vi "AutoAlign_P541_V2.vi"() -> ()   [LabVIEW 2014]
uses:
  Controls/StageStates.ctl
  Controls/GraphNotifier2D.ctl
panel:
  out "Current Step":i32
  in  "Done":bool
  in  "Repeat":bool
  in  "Start":bool
  out "Cursor Position":dbl=40.46
  in  "InitialStep":dbl=-0.5
  in  "StepSize":dbl=0.03
  in  "Number Of Steps":i32=45
  out "Intensity Graph":sgl[][](graph)=[[1726.0, 1806.0, 1623.0, 1740.0, 1902.0, 2025.0, 2061.0, 2397.0, 1982.0, 2142.0, 1921.0, 1825.0, 1807.0, 1676.0, 1719.0], [1834.0, 1961.0, 1598.0, 2017.0, 2102.0, 2328.0, 2583.0, 2454.0, 2515.0, 2699.0, 2220.0, 2038.0, 1897.0, 1896.0, 1808.0], [1796.0, 1929.0, 2014.0, 2227.0, 2672.0, 3226.0, 3334.0, 3386.0, 3268.0, 2996.0, 2332.0, 2163.0, 1901.0, 1735.0, 1698.0], [1808.0, 2338.0, 2431.0, 2752.0, 3453.0, 4017.0, 4563.0, 4369.0, 4047.0, 3273.0, 2724.0, 2242.0, 2046.0, 1830.0, 1856.0], [1912.0, 2124.0, 3081.0, 2979.0, 5386.0, 11058.0, 13706.0, 11119.0, 6549.0, 3853.0, 2769.0, 2421.0, 1921.0, 1945.0, 1667.0], [1802.0, 2329.0, 2974.0, 5101.0, 13243.0, 29557.0, 37323.0, 29866.0, 11701.0, 4217.0, 2995.0, 2488.0, 2124.0, 2138.0, 1748.0], [1855.0, 2667.0, 2858.0, 6518.0, 22689.0, 47134.0, 57757.0, 40932.0, 16892.0, 4794.0, 2975.0, 2648.0, 2316.0, 1940.0, 2196.0], [1840.0, 2513.0, 2969.0, 6113.0, 20925.0, 44575.0, 52306.0, 35893.0, 13438.0, 3959.0, 2980.0, 2333.0, 2128.0, 1717.0, 1820.0], [1975.0, 2578.0, 2513.0, 4337.0, 10762.0, 22714.0, 27719.0, 17796.0, 6495.0, 3198.0, 2732.0, 2148.0, 1973.0, 1982.0, 1689.0], [1678.0, 2147.0, 2574.0, 2995.0, 4337.0, 7306.0, 8045.0, 5820.0, 3423.0, 2628.0, 2656.0, 2059.0, 2116.0, 1972.0, 1626.0], [1892.0, 2079.0, 2546.0, 2756.0, 2841.0, 3166.0, 3141.0, 2947.0, 2684.0, 2415.0, 1923.0, 1806.0, 2081.0, 1695.0, 1756.0], [1617.0, 1885.0, 1958.0, 2510.0, 2675.0, 2479.0, 2435.0, 2624.0, 2645.0, 2107.0, 1819.0, 2019.0, 1839.0, 1623.0, 1670.0], [1609.0, 1896.0, 1887.0, 1962.0, 2214.0, 2352.0, 2290.0, 2047.0, 1815.0, 2022.0, 1883.0, 1801.0, 1521.0, 1615.0, 1723.0], [1697.0, 1808.0, 1977.0, 1969.0, 2042.0, 1988.0, 2305.0, 2063.0, 1959.0, 1814.0, 1844.0, 1590.0, 1578.0, 1755.0, 1573.0], [1645.0, 1684.0, 1821.0, 1765.0, 1973.0, 1906.0, 2005.0, 1822.0, 1736.0, 1850.0, 1649.0, 1802.0, 1476.0, 1658.0, 1637.0]]
  in  "Quit":bool
  out "Sample":cluster{dbl[], dbl[]}[](graph)
  in  "Accumulations":i32=10
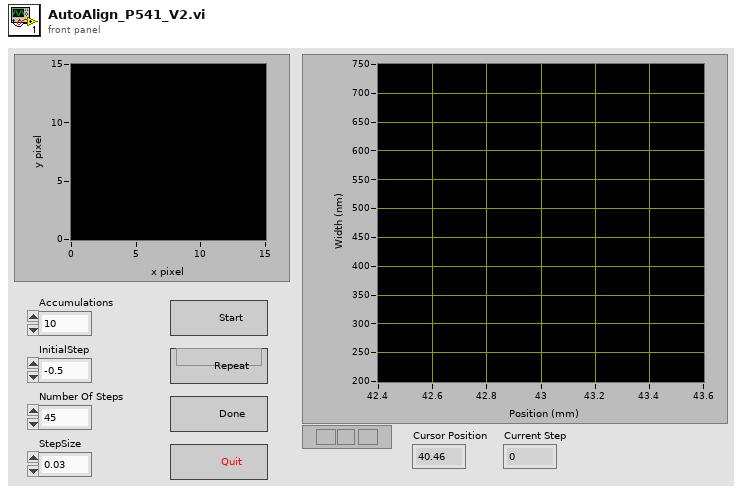
[diagram p1: front panel]
types:
  T1 = typedef "GraphNotifier2D.ctl" = cluster{"Xpos":i32, "Ypos":i32, "subarray":sgl[][], "Intensity":sgl}
  T2 = typedef "LabVIEW Interface for Arduino.lvlib/Arduino Resource.ctl" = cluster{"VISA resource":refnum<visa-resource-name>, "Board Type":T3, "Connection Type":enum8{"USB / Serial"}, "Bytes Per Packet (15)":u8}
  T3 = typedef "LabVIEW Interface for Arduino.lvlib/Board Type.ctl" = enum16{"Uno", "Dimuelanove w/Atmega 328", "Mega 2560"}
  T4 = typedef "StageStates.ctl" = enum16{"POSITION", "MVR", "MOVE", "HALT", "ONTARGET", "ERROR", "EXIT", "HOME", "ZEROPOS", "NANOPOS", "QUIT", "ANALOG"}
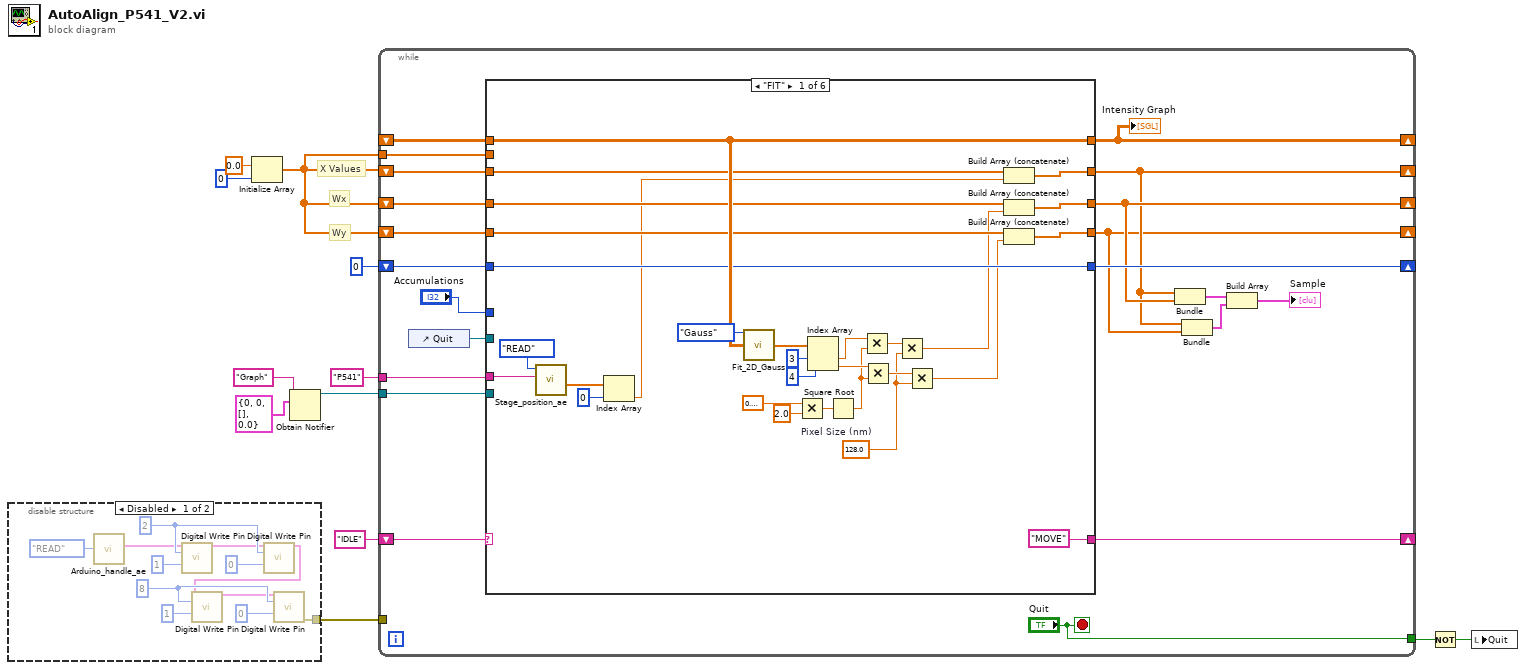
[diagram p0: block diagram]
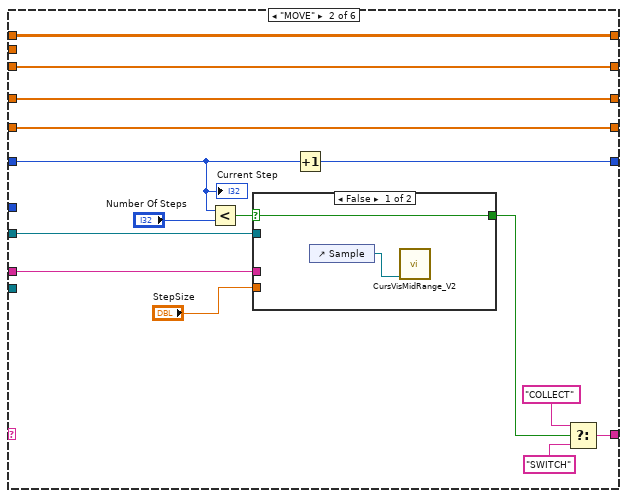
[diagram p3: hidden frame]
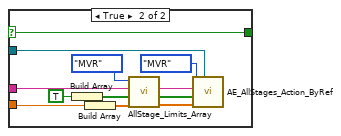
[diagram p4: hidden frame]
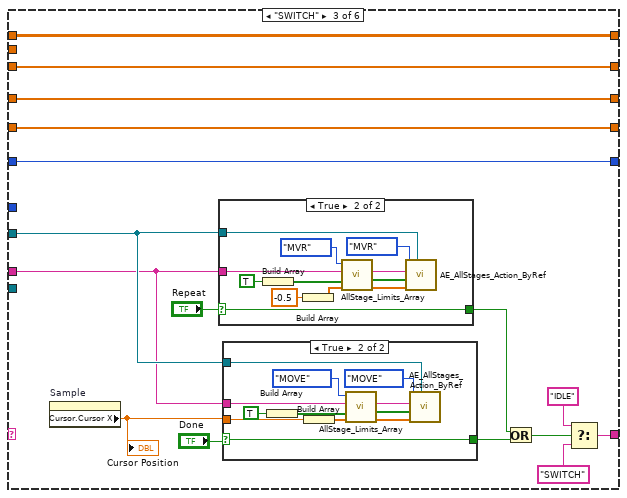
[diagram p5: hidden frame]
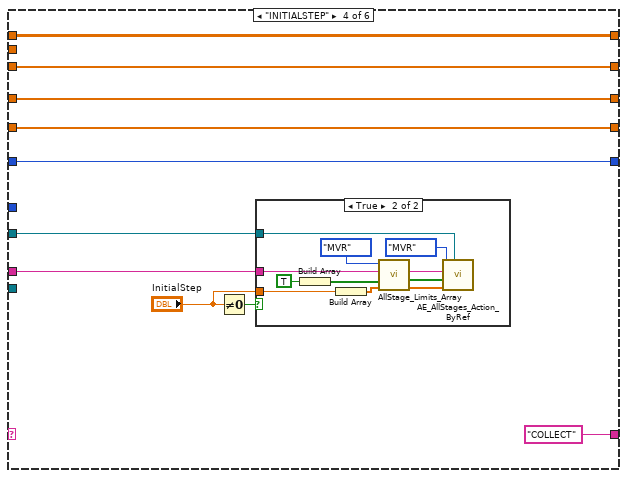
[diagram p8: hidden frame]
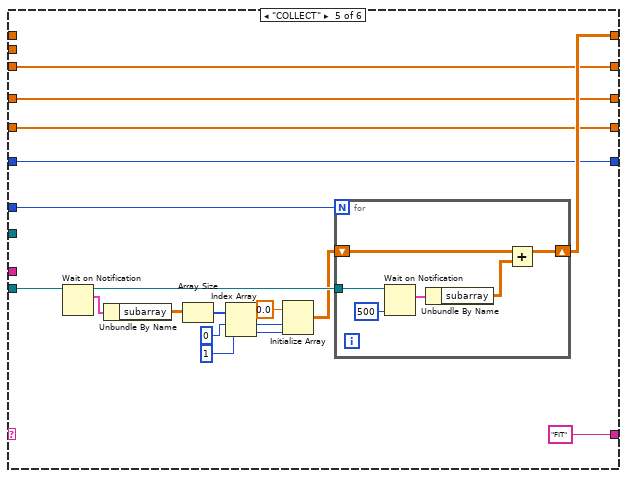
[diagram p10: hidden frame]
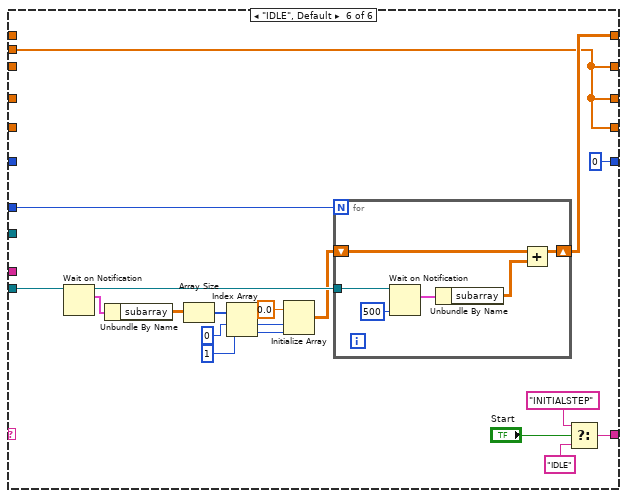
[diagram p11: hidden frame]
diagram:
  # "Wy"
  # "Wx"
  # "X Values"
  n1 = disable-structure shown="Disabled" {
    disable-tunnel: [w13 _] -> w9
    frame Disabled {
      w24 = u8 8 ("Digital I/O Pin (0)")
      w19 = u8 2 ("Digital I/O Pin (0)")
      n2 = call "Arduino_handle_ae.vi"("Enum"=enum16{"WRITE", "READ"}."READ") -> ("Arduino Resource Out"=w18:T2)  [unwired: 10 in]
      n3 = call <vilib>:"Digital Write Pin.vi"("Arduino Resource"=w18, "Digital I/O Pin (0)"=w19, "Value (0)"=u8 1) -> ("Arduino Resource"=w14:T2)  [unwired: 11 in, 1 out]
      n4 = call <vilib>:"Digital Write Pin.vi"("Arduino Resource"=w14, "Digital I/O Pin (0)"=w19, "Value (0)"=u8 0) -> ("Arduino Resource"=w23:T2)  [unwired: 11 in, 1 out]
      n5 = call <vilib>:"Digital Write Pin.vi"("Arduino Resource"=w23, "Digital I/O Pin (0)"=w24, "Value (0)"=u8 1) -> ("Arduino Resource"=w22:T2)  [unwired: 11 in, 1 out]
      n6 = call <vilib>:"Digital Write Pin.vi"("Arduino Resource"=w22, "Digital I/O Pin (0)"=w24, "Value (0)"=u8 0) -> ("error out"=w13:errorcluster)  [unwired: 11 in, 1 out]
    }
    frame Enabled {
    }
  }
  n7 = Initialize Array(0.0 ("element"), 0 ("dimension size")) -> (w1:dbl[])
  n8 = Obtain Notifier(name (unnamed)="Graph", notification data type=T1 {"Xpos"=0, "Ypos"=0, "subarray"=[], "Intensity"=0.0}) -> (notifier out=w6:refnum<notifier>)  [unwired: 2 in, 2 out]
  n9 = while {
    shift-right: [w44] -> _
    shift-left: _ -> [w45]
    shift-right: [w29] -> _
    shift-left: w1 -> [w35]
    shift-right: [w43] -> _
    shift-left: "IDLE" -> [w39]
    shift-right: [w41] -> _
    shift-left: 0 ("NumberOfSteps 2") -> [w42]
    tunnel: w6 -> [w38]
    tunnel: "P541" ("StageID") -> [w36]
    tunnel: w9 -> [_]
    tunnel: ["Quit"] -> w5
    shift-right: [w30] -> _
    shift-left: w1 -> [w33]
    shift-right: [w28] -> _
    shift-left: w1 -> [w32]
    tunnel: w1 -> [w31]
    stop <- "Quit" stop-if-true
    n10 = control-ref of="Quit"() -> (w40:refnum<vi>)
    n11 = case shown="\"FIT\"" w39 {
      tunnel: [w73 w89 w118 w155 w184 w209] -> w44
      tunnel: w45 -> [w73 w89 w118 w155 _ _]
      tunnel: w35 -> [w54 w77 w106 w148 w169 _]
      tunnel: w36 -> [w70 w80 w115 w151 _ _]
      tunnel: ["MOVE" w86 w112 "COLLECT" "FIT" w207] -> w43
      tunnel: w42 -> [w71 w84 w119 w154 w183 _]
      tunnel: [w71 w85 w119 w154 w183 0 ("NumberOfSteps 2")] -> w41
      tunnel: w40 -> [_ w82 w117 w153 _ _]
      tunnel: w38 -> [_ _ _ _ w172 w201]
      tunnel: "Accumulations" -> [_ _ _ _ w181 w204]
      tunnel: w33 -> [w52 w76 w105 w147 w168 _]
      tunnel: w32 -> [w53 w75 w104 w146 w167 _]
      tunnel: [w51 w77 w106 w148 w169 w191] -> w29
      tunnel: [w50 w76 w105 w147 w168 w191] -> w30
      tunnel: [w49 w75 w104 w146 w167 w191] -> w28
      tunnel: w31 -> [_ _ _ _ _ w191]
      frame "FIT" {
        w55 = 128.0  # Pixel Size (nm)
        n12 = call "Stage_position_ae.vi"("StageID"=w70, "Enum"=enum16{"WRITE", "READ"}."READ") -> ("Position Out"=w63:dbl[])  [unwired: 8 in, 1 out]
        n13 = Index Array(array=w63, index=0) -> (element=w48:dbl)
        n14 = call "Fit_2D_Gauss.vi"("Enum"=enum16{"Gauss", "Lorentz"}."Gauss", "Image IN"=w73) -> ("Fit Parameters"=w74:dbl[])  [unwired: 12 in, 1 out]
        n15 = Multiply(x=0.6931471805599453, y=2.0) -> (x*y=w67:dbl)
        n16 = Index Array(array=w74, index #1=3 ("index"), index #2=4 ("index")) -> (element #1=w66:dbl, element #2=w58:dbl)
        n17 = Square Root(x=w67) -> (sqrt(x)=w57:dbl)
        n18 = Multiply(x=w66, y=w57) -> (x*y=w59:dbl)
        n19 = Multiply(x=w58, y=w57) -> (x*y=w56:dbl)
        n20 = Multiply(x=w59, y=w55) -> (x*y=w47:dbl)
        n21 = Multiply(x=w56, y=w55) -> (x*y=w46:dbl)
        n22 = Build Array (concatenate)(w54, w48) -> (w51:dbl[])
        n23 = Build Array (concatenate)(w52, w47) -> (w50:dbl[])
        n24 = Build Array (concatenate)(w53, w46) -> (w49:dbl[])
      }
      frame "MOVE" {
        n25 = Less?(x=w84, y="Number Of Steps") -> (x < y?=w78:bool)
        n26 = case shown="False" w78 {
          selector: w78 -> [w91 w100]
          tunnel: w80 -> [_ w95]
          tunnel: w82 -> [_ w101]
          tunnel: [w91 w100] -> w83
          tunnel: "StepSize" -> [_ w93]
          frame False {
            n27 = control-ref of="Sample"() -> (w90:refnum<vi>)
            n28 = call "CursVisMidRange_V2.vi"("Sample 2"=w90) -> ()  [unwired: 11 in]
          }
          frame True {
            n29 = Build Array(TRUE) -> (w96:bool[])
            n30 = Build Array(w93) -> (w92:dbl[])
            n31 = call "AllStage_Limits_Array.vi"("Step(um)/Position(units)"=w92, "Axis"=w96, "Stage ID"=w95, "MOVE/MVR"=enum16{"MOVE", "MVR"}."MVR") -> ("Positions"=w97:dbl[], "Boolean Array"=w98:bool[], "Stage ID"=w99:string)  [unwired: 5 in]
            n32 = call "AE_AllStages_Action_ByRef.vi"("Abort"=w101, "Positions"=w97, "Axis"=w98, "Stage ID"=w99, "Action"=StageStates."MVR") -> ()  [unwired: 3 in, 4 out]
          }
        }
        n33 = Increment(x=w84) -> (x+1=w85:i32)
        n34 = Select(t="COLLECT", s=w83, f="SWITCH") -> (s? t:f=w86:string)
        "Current Step" <- w84
      }
      frame "SWITCH" {
        n35 = property on="Sample" class="XYGraph (strict)"() -> ("Cursor.Cursor X"=w116:dbl)  [unwired: 2 in, 2 out]
        "Cursor Position" <- w116
        n36 = case shown="True" "Repeat" {
          selector: "Repeat" -> [w133 w135]
          tunnel: w115 -> [_ w136]
          tunnel: w117 -> [_ w143]
          tunnel: [w133 w135] -> w108
          frame False {
          }
          frame True {
            n37 = Build Array(TRUE) -> (w141:bool[])
            n38 = Build Array(-0.5 ("Step(um)/Position(units)")) -> (w134:dbl[])
            n39 = call "AllStage_Limits_Array.vi"("Step(um)/Position(units)"=w134, "Axis"=w141, "Stage ID"=w136, "MOVE/MVR"=enum16{"MOVE", "MVR"}."MVR") -> ("Positions"=w138:dbl[], "Boolean Array"=w139:bool[], "Stage ID"=w140:string)  [unwired: 5 in]
            n40 = call "AE_AllStages_Action_ByRef.vi"("Abort"=w143, "Positions"=w138, "Axis"=w139, "Stage ID"=w140, "Action"=StageStates."MVR") -> ()  [unwired: 3 in, 4 out]
          }
        }
        n41 = case shown="True" "Done" {
          selector: "Done" -> [w120 w122]
          tunnel: w115 -> [_ w123]
          tunnel: w117 -> [_ w130]
          tunnel: w116 -> [_ w124]
          tunnel: [w120 w122] -> w107
          frame False {
          }
          frame True {
            n42 = Build Array(TRUE) -> (w128:bool[])
            n43 = Build Array(w124) -> (w121:dbl[])
            n44 = call "AllStage_Limits_Array.vi"("Step(um)/Position(units)"=w121, "Axis"=w128, "Stage ID"=w123, "MOVE/MVR"=enum16{"MOVE", "MVR"}."MOVE") -> ("Positions"=w125:dbl[], "Boolean Array"=w126:bool[], "Stage ID"=w127:string)  [unwired: 5 in]
            n45 = call "AE_AllStages_Action_ByRef.vi"("Abort"=w130, "Positions"=w125, "Axis"=w126, "Stage ID"=w127, "Action"=StageStates."MOVE") -> ()  [unwired: 3 in, 4 out]
          }
        }
        n46 = Or(x=w108, y=w107) -> (x .or. y?=w111:bool)
        n47 = Select(t="IDLE", s=w111, f="SWITCH") -> (s? t:f=w112:string)
      }
      frame "INITIALSTEP" {
        n48 = Not Equal To 0?(x="InitialStep") -> (x != 0?=w150:bool)
        n49 = case shown="True" w150 {
          tunnel: w151 -> [_ w162]
          tunnel: w153 -> [_ w164]
          tunnel: "InitialStep" -> [_ w163]
          frame False {
          }
          frame True {
            n50 = Build Array(TRUE) -> (w160:bool[])
            n51 = Build Array(w163) -> (w156:dbl[])
            n52 = call "AllStage_Limits_Array.vi"("Step(um)/Position(units)"=w156, "Axis"=w160, "Stage ID"=w162, "MOVE/MVR"=enum16{"MOVE", "MVR"}."MVR") -> ("Positions"=w157:dbl[], "Boolean Array"=w158:bool[], "Stage ID"=w159:string)  [unwired: 5 in]
            n53 = call "AE_AllStages_Action_ByRef.vi"("Abort"=w164, "Positions"=w157, "Axis"=w158, "Stage ID"=w159, "Action"=StageStates."MVR") -> ()  [unwired: 3 in, 4 out]
          }
        }
      }
      frame "COLLECT" {
        n54 = Wait on Notification(notifier=w172) -> (notifier out=w171:refnum<notifier>, notification=w180:T1)  [unwired: 3 in, 2 out]
        n55 = Unbundle By Name(w180) -> ("subarray"=w179:sgl[][])
        n56 = Array Size(array=w179) -> (size(s)=w178:i32[])
        n57 = Index Array(array=w178, index #1=0 ("index"), index #2=1 ("index")) -> (element #1=w175:i32, element #2=w174:i32)
        n58 = Initialize Array(sgl 0.0 ("element"), w175, w174) -> (w170:sgl[][])
        n59 = for {
          N: w181 -> [_]
          shift-right: [w190] -> w184
          shift-left: w170 -> [w189]
          tunnel: w171 -> [w187]
          n60 = Wait on Notification(notifier=w187, timeout in ms (-1)=500) -> (notification=w186:T1)  [unwired: 2 in, 3 out]
          n61 = Unbundle By Name(w186) -> ("subarray"=w185:sgl[][])
          n62 = Add(x=w189, y=w185) -> (x+y=w190:sgl[][])
        }
      }
      frame "IDLE", Default {
        n63 = Wait on Notification(notifier=w201) -> (notifier out=w200:refnum<notifier>, notification=w203:T1)  [unwired: 3 in, 2 out]
        n64 = Unbundle By Name(w203) -> ("subarray"=w202:sgl[][])
        n65 = Array Size(array=w202) -> (size(s)=w199:i32[])
        n66 = Index Array(array=w199, index #1=0 ("index"), index #2=1 ("index")) -> (element #1=w196:i32, element #2=w195:i32)
        n67 = Initialize Array(sgl 0.0 ("element"), w196, w195) -> (w193:sgl[][])
        n68 = for {
          N: w204 -> [_]
          shift-right: [w215] -> w209
          shift-left: w193 -> [w214]
          tunnel: w200 -> [w212]
          n69 = Wait on Notification(notifier=w212, timeout in ms (-1)=500) -> (notification=w211:T1)  [unwired: 2 in, 3 out]
          n70 = Unbundle By Name(w211) -> ("subarray"=w210:sgl[][])
          n71 = Add(x=w214, y=w210) -> (x+y=w215:sgl[][])
        }
        n72 = Select(t="INITIALSTEP", s="Start", f="IDLE") -> (s? t:f=w207:string)
      }
    }
    "Intensity Graph" <- w44
    n73 = Bundle(w29, w30) -> (w27:cluster{dbl[], dbl[]})  [unwired: 1 in]
    n74 = Bundle(w29, w28) -> (w26:cluster{dbl[], dbl[]})  [unwired: 1 in]
    n75 = Build Array(w27, w26) -> (→"Sample":cluster{dbl[], dbl[]}[])
  }
  n76 = Not(x=w5) -> (.not. x?=w4:bool)
  n77 = local write "Quit"(w4) -> ()
